vi "Write User Source Signal.vi"(0 "signal index":u16, 2 "shared":refnum<class "niUSRP Rx Core v1 FPGA.lvclass">=refnum, 9 "pre-conditioned signal":bool) -> ()   [LabVIEW 2023, in "niUSRP Rx Core v1 FPGA.lvclass"]
doc: "this VI writes a UserSource signal to Routing, which can be configured from the host (e.g. - /deviceAlias/UserSource0 )."
uses:
  <instrlib>/niUSRP/Reference FPGA/Rx Core/niUSRP Rx Core v1 FPGA.lvclass
  <instrlib>/niVST/Reference FPGA/FPGA/Routing/v1/Base/niVST Routing (Base) v1 FPGA.lvclass
  <instrlib>/niVST/Reference FPGA/FPGA/niUSRP Rx Core v1 FPGA/niUSRP Rx Core v1 FPGA.lvclass
  <instrlib>/niVST/Reference FPGA/FPGA/Routing/v1/Base/Public/Typedefs/User Source Signal.ctl
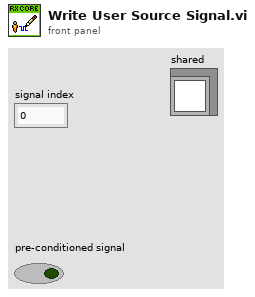
[diagram p1: front panel]
types:
  T1 = typedef "niVST Routing (Base) v1 FPGA.lvclass/User Source Signal.ctl" = enum16{"UserSource0", "UserSource1", "UserSource2", "UserSource3", "UserSource4", "UserSource5", "UserSource6", "UserSource7"}
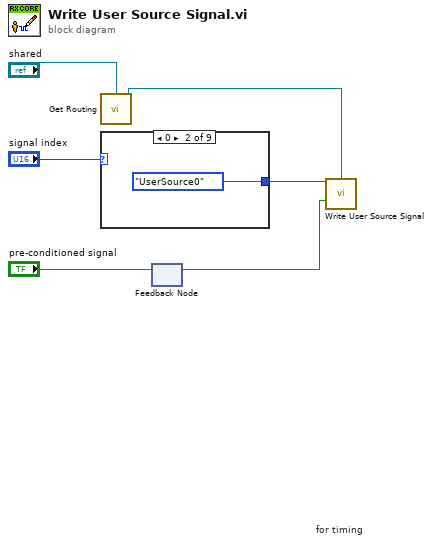
[diagram p0: block diagram]
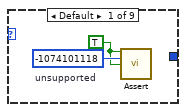
[diagram p2: hidden frame]
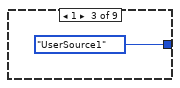
[diagram p3: hidden frame]
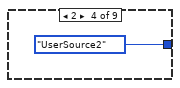
[diagram p4: hidden frame]
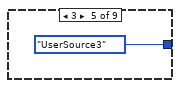
[diagram p5: hidden frame]
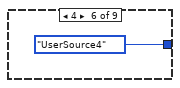
[diagram p6: hidden frame]
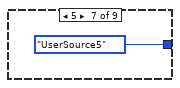
[diagram p7: hidden frame]
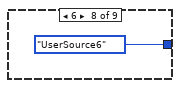
[diagram p8: hidden frame]
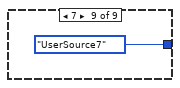
[diagram p9: hidden frame]
diagram:
  n1 = call-dynamic "Get Routing.vi"("shared"="shared") -> ("routing"=w4:refnum<class "niVST Routing (Base) v1 FPGA.lvclass">)  [unwired: 14 in]
  n2 = case shown="0" "signal index" {
    tunnel: [_ User_Source_Signal."UserSource0" ("signal select") User_Source_Signal."UserSource1" ("signal select") User_Source_Signal."UserSource2" ("signal select") User_Source_Signal."UserSource3" ("signal select") User_Source_Signal."UserSource4" ("signal select") User_Source_Signal."UserSource5" ("signal select") User_Source_Signal."UserSource6" ("signal select") User_Source_Signal."UserSource7" ("signal select")] -> w3
    frame Default {
      w7 = TRUE ("assert")
      w8 = -1074101118  # unsupported
      n3 = call <instrlib>:"Assert.vi"("assert"=w7, "error code"=w8, "enable show error"=w7) -> ()  [unwired: 13 in]
    }
    frame 0 {
    }
    frame 1 {
    }
    frame 2 {
    }
    frame 3 {
    }
    frame 4 {
    }
    frame 5 {
    }
    frame 6 {
    }
    frame 7 {
    }
  }
  n4 = feedback-in #1("pre-conditioned signal") -> ()
  n5 = feedback #1 "for timing"() -> (w1:bool)  [unwired: 1 in]
  n6 = call-dynamic "Write User Source Signal.vi"("signal select"=w3, "routing (Base)"=w4, "pre-conditioned signal"=w1) -> ()  [unwired: 13 in]
